vi "libssh2_channel_forward_accept.vi"(8 "error in (no error)":errorcluster, 11 "listener":T2) -> (0 "error out":errorcluster, 3 "channel":T1)   [LabVIEW 2013, in "libssh2.lvlib"]
doc: "Accept a forwarded connection on a listening channel."
uses:
  libssh2.lvlib
  Listener Refnum.ctl
  Channel Refnum.ctl
  Acquire Session.vi
  Release Session.vi
  Not A Listener.vi
  <vilib>/Utility/error.llb/Error Cluster From Error Code.vi
  Global Settings.vi
  Read Session Refnum.vi
  <vilib>/Utility/semaphor.llb/Acquire Semaphore.vi
  <vilib>/Utility/semaphor.llb/Release Semaphore.vi
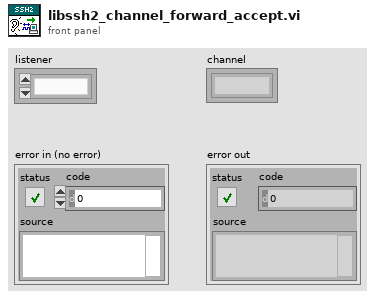
[diagram p1: front panel]
types:
  T1 = typedef "libssh2.lvlib/Channel Refnum.ctl" = refnum<k1>
  T2 = typedef "libssh2.lvlib/Listener Refnum.ctl" = refnum<k1>
  T3 = typedef "libssh2.lvlib/Session Refnum.ctl" = refnum<k1>
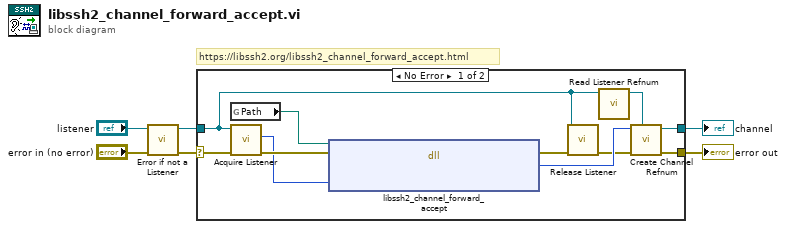
[diagram p0: block diagram]
diagram:
  # "https://libssh2.org/libssh2_channel_forward_accept.html"
  n1 = call "Error if not a Listener.vi"("error in (no error)"="error in (no error)", "listener"="listener") -> ("error out"=w3:errorcluster, "listener out"=w1:T2)  [unwired: 8 in]
  n2 = case shown="No Error" w3 {
    selector: w3 -> [w11 w18]
    tunnel: [w16 w18] -> w6
    tunnel: [w14 _] -> w5
    tunnel: w1 -> [w7 _]
    frame No Error {
      n3 = global read "Global Settings.vi" "Path"() -> (w10:path)
      n4 = call "Acquire Listener.vi"("error in (no error)"=w11, "listener"=w7) -> ("error out"=w13:errorcluster, "LIBSSH2_LISTENER*"=w12:u64)  [unwired: 8 in]
      n5 = dll-call lib="?" fn="libssh2_channel_forward_accept"(path in=w10, error in=w13, "listener"=w12) -> (error out=w17:errorcluster, "return value"=w15:u64)  [unwired: 2 in, 1 out]
      n6 = call "Release Listener.vi"("error in (no error)"=w17, "listener"=w7) -> ("error out"=w9:errorcluster)  [unwired: 9 in]
      n7 = call "Read Listener Refnum.vi"("listener"=w7) -> ("session"=w8:T3)  [unwired: 8 in, 2 out]
      n8 = call "Create Channel Refnum.vi"("session"=w8, "error in (no error)"=w9, "LIBSSH2_CHANNEL*"=w15) -> ("error out"=w16:errorcluster, "channel"=w14:T1)  [unwired: 7 in]
    }
    frame Error {
    }
  }
  "error out" <- w6
  "channel" <- w5
